vi "FindBuildSpecs.vi"(8 "error in (no error)":errorcluster, 11 "ExecuteMultipleBuildSpecs in":refnum<class "ExecuteMultipleBuildSpecs.lvclass">) -> (0 "error out":errorcluster, 3 "ExecuteMultipleBuildSpecs out":refnum<class "ExecuteMultipleBuildSpecs.lvclass">)   [LabVIEW 2014, in "ExecuteMultipleBuildSpecs.lvclass"]
doc: "Finds all build specs in the provided project that match the criteria for the multiple build spec operation."
uses:
  ExecuteMultipleBuildSpecs.lvclass
  SpecInformation.ctl
  ExecuteMultipleBuildSpecs.lvclass/ExecuteMultipleBuildSpecs.ctl
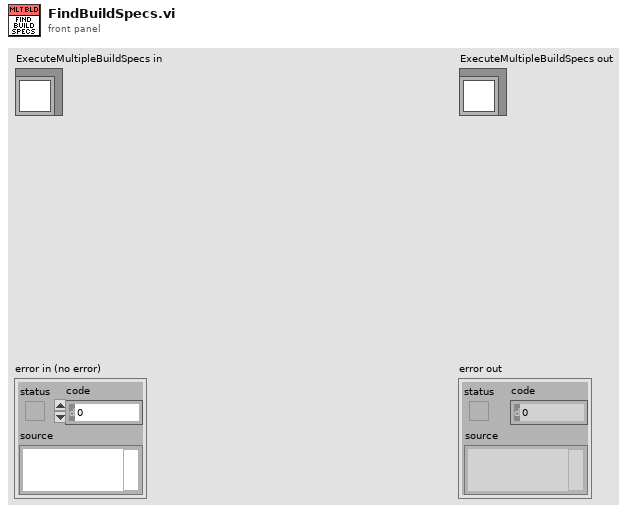
[diagram p1: front panel]
types:
  T1 = typedef "ExecuteMultipleBuildSpecs.lvclass/SpecInformation.ctl" = cluster{"Target":string, "Build Spec":string}
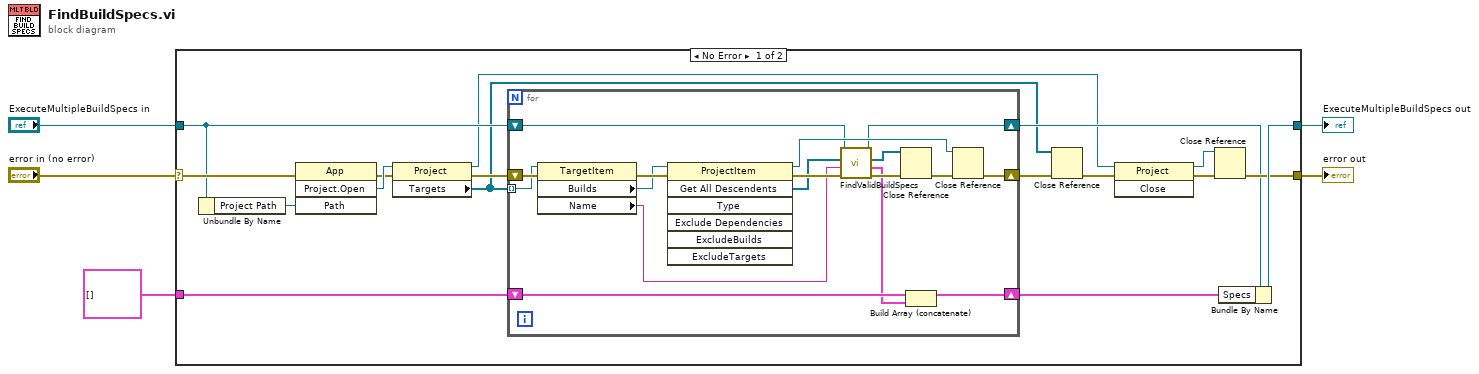
[diagram p0: block diagram]
diagram:
  n1 = case shown="No Error" "error in (no error)" {
    selector: "error in (no error)" -> [w17 w41]
    tunnel: [w18 w41] -> w4
    tunnel: [w21 w40] -> w2
    tunnel: "ExecuteMultipleBuildSpecs in" -> [w9 w40]
    tunnel: T1[] [] -> [w11 _]
    frame No Error {
      n2 = Unbundle By Name(w9) -> ("Project Path"=w22:path)
      n3 = invoke class="App" method="Project.Open"(error in=w17, "Path"=w22) -> (error out=w12:errorcluster, "Project:Open"=w14:refnum<vi>)  [unwired: 2 in, 2 out]
      n4 = property class="Project"(reference=w14, error in=w12) -> (reference out=w6:refnum<vi>, error out=w16:errorcluster, "Targets"=w7:refnum<vi>[])
      n5 = for {
        tunnel: w7 -> [w38] mode=indexing
        shift-right: [w32] -> w15
        shift-left: w16 -> [w39]
        shift-right: [w34] -> w10
        shift-left: w11 -> [w35]
        shift-right: [w23] -> w8
        shift-left: w9 -> [w24]
        n6 = property class="TargetItem"(reference=w38, error in=w39) -> (error out=w37:errorcluster, "Builds"=w36:refnum<vi>, "Name"=w28:string)  [unwired: 1 out]
        n7 = invoke class="ProjectItem" method="Get All Descendents"(reference=w36, error in=w37) -> (reference out=w31:refnum<vi>, error out=w30:errorcluster, "All Descendents"=w29:refnum<vi>[])  [unwired: 5 in, 4 out]
        n8 = call-dynamic "FindValidBuildSpecs.vi"("error in (no error)"=w30, "Target Name"=w28, "ProjectItem Refnums"=w29, "ExecuteMultipleBuildSpecs in"=w24) -> ("error out"=w27:errorcluster, "Specs"=w26:T1[], "dup ProjectItem Refnums"=w25:refnum<vi>[], "ExecuteMultipleBuildSpecs out"=w23:refnum<class "ExecuteMultipleBuildSpecs.lvclass">)  [unwired: 4 in]
        n9 = Close Reference(reference=w25, error in (no error)=w27) -> (error out=w33:errorcluster)
        n10 = Build Array (concatenate)(w35, w26) -> (w34:T1[])
        n11 = Close Reference(reference=w31, error in (no error)=w33) -> (error out=w32:errorcluster)
      }
      n12 = Close Reference(reference=w7, error in (no error)=w15) -> (error out=w13:errorcluster)
      n13 = invoke class="Project" method="Close"(reference=w6, error in=w13) -> (reference out=w19:refnum<vi>, error out=w20:errorcluster)  [unwired: 1 in, 1 out]
      n14 = Close Reference(reference=w19, error in (no error)=w20) -> (error out=w18:errorcluster)
      n15 = Bundle By Name(cluster=w8, "Specs"=w10) -> (w21:refnum<class "ExecuteMultipleBuildSpecs.lvclass">)
    }
    frame Error {
    }
  }
  "error out" <- w4
  "ExecuteMultipleBuildSpecs out" <- w2
